vi "Manager QueryPluginTypes.vi"(6 "contextId":T1, 8 "error in":errorcluster, 9 "timeout (ms)":i32=-1, 10 "Request Data":T6, 11 "gRPC ID":T1) -> (0 "error out":errorcluster, 2 "Response Data":T2, 3 "gRPC ID out":T1)   [LabVIEW 2021, in "CIF_Manager_client.lvlib"]
uses:
  CIF_Manager_client.lvlib
  14035477-4c25-4107-8ed5-d0c4ef420ce5.vi
  RPC Messages/cif_common_ShortVersion_Flat.ctl
  RPC Messages/cif_management_common_PluginMetadata_Flat.ctl
  RPC Messages/cif_manager_PluginType_Flat.ctl
  RPC Messages/cif_manager_QueryPluginTypesResponse_Flat.ctl
  <vilib>/gRPC/LabVIEW gRPC Library/Shared/grpcId.ctl
  <vilib>/gRPC/LabVIEW gRPC Library/grpc-lvsupport-release.lvlib
  RPC Messages/cif_management_common_PluginMetadata.ctl
  RPC Messages/cif_common_ShortVersion.ctl
  RPC Messages/cif_manager_PluginType.ctl
  RPC Messages/cif_manager_QueryPluginTypesResponse.ctl
  RPC Messages/cif_manager_QueryPluginTypesRequest.ctl
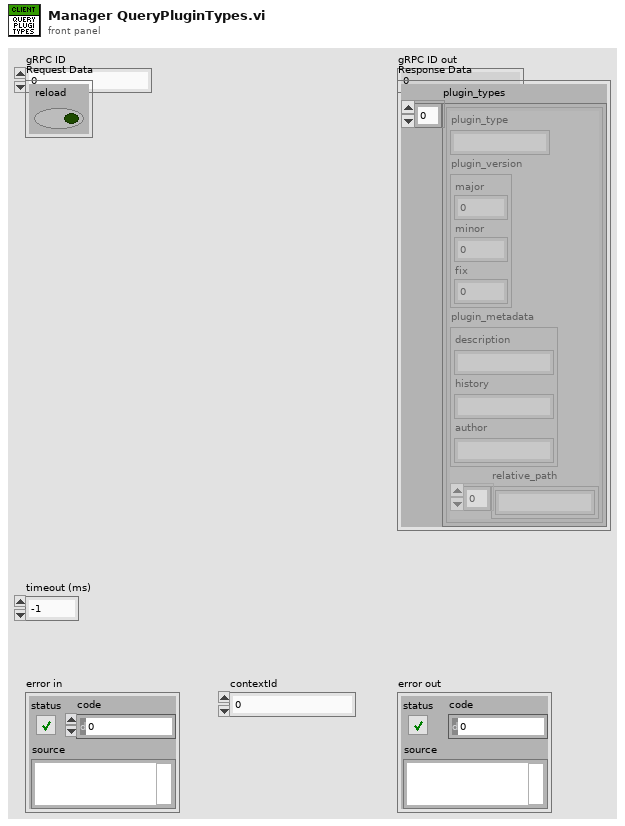
[diagram p1: front panel]
types:
  T1 = typedef "grpc-lvsupport-release.lvlib/grpcId.ctl" = u64
  T2 = typedef "CIF_Manager_client.lvlib/cif_manager_QueryPluginTypesResponse.ctl" = cluster{"plugin_types":T3[]}
  T3 = typedef "CIF_Manager_client.lvlib/cif_manager_PluginType.ctl" = cluster{"plugin_type":string, "plugin_version":T4, "plugin_metadata":T5, "relative_path":string[]}
  T4 = typedef "CIF_Manager_client.lvlib/cif_common_ShortVersion.ctl" = cluster{"major":u32, "minor":u32, "fix":u32}
  T5 = typedef "CIF_Manager_client.lvlib/cif_management_common_PluginMetadata.ctl" = cluster{"description":string, "history":string, "author":string}
  T6 = typedef "CIF_Manager_client.lvlib/cif_manager_QueryPluginTypesRequest.ctl" = cluster{"reload":bool}
  T7 = typedef "CIF_Manager_client.lvlib/cif_manager_QueryPluginTypesResponse_Flat.ctl" = cluster{"plugin_types":T8[]}
  T8 = typedef "CIF_Manager_client.lvlib/cif_manager_PluginType_Flat.ctl" = cluster{"plugin_type":string, "plugin_version":T9, "plugin_metadata":T10, "relative_path":string[]}
  T9 = typedef "CIF_Manager_client.lvlib/cif_common_ShortVersion_Flat.ctl" = cluster{"major":u32, "minor":u32, "fix":u32}
  T10 = typedef "CIF_Manager_client.lvlib/cif_management_common_PluginMetadata_Flat.ctl" = cluster{"description":string, "history":string, "author":string}
  T11 = typedef "CIF_Manager_client.lvlib/cif_manager_QueryPluginTypesRequest_Flat.ctl" = cluster{"reload":bool}
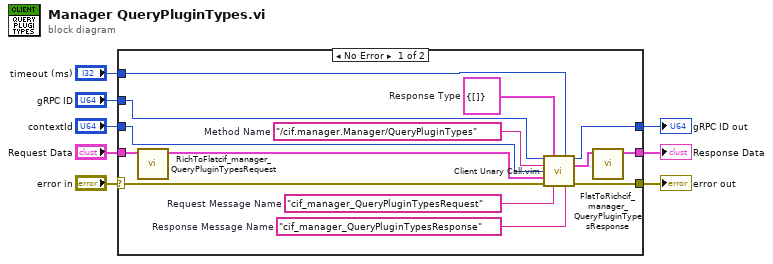
[diagram p0: block diagram]
diagram:
  n1 = case shown="No Error" "error in" {
    selector: "error in" -> [w18 w23]
    tunnel: [w17 w23] -> w7
    tunnel: "gRPC ID" -> [w16 w24]
    tunnel: [w15 w24] -> w5
    tunnel: "Request Data" -> [w12 _]
    tunnel: [w9 _] -> w3
    tunnel: "timeout (ms)" -> [w14 _]
    tunnel: "contextId" -> [w13 _]
    frame No Error {
      w19 = "cif_manager_QueryPluginTypesResponse"  # Response Message Name
      w20 = "cif_manager_QueryPluginTypesRequest"  # Request Message Name
      w21 = T7 {"plugin_types"=[]}  # Response Type
      w22 = "/cif.manager.Manager/QueryPluginTypes"  # Method Name
      n2 = call "RichToFlatcif_manager_QueryPluginTypesRequest.vi"("InputCluster"=w12) -> ("OutputCluster"=w11:T11)  [unwired: 10 in]
      n3 = call "Client Unary Call.vim"("ClientID in"=w16, "Response Type"=w21, "timeout (ms)"=w14, "Method Name"=w22, "contextId"=w13, "Request Data"=w11, "error in"=w18, "Request Message Name"=w20, "Response Message Name"=w19) -> ("ClientID out"=w15:u64, "Response Data"=w10:T7, "error out"=w17:errorcluster)  [unwired: 4 in]
      n4 = call "FlatToRichcif_manager_QueryPluginTypesResponse.vi"("InputCluster"=w10) -> ("OutputCluster"=w9:T2)  [unwired: 10 in]
    }
    frame Error {
    }
  }
  "error out" <- w7
  "gRPC ID out" <- w5
  "Response Data" <- w3
